vi "getSelfNode.vi"(8 "error in (no error)":errorcluster, 11 "Node in":refnum<class "Node.lvclass">) -> (0 "error out":errorcluster, 2 "selfNode":refnum<data-value>, 3 "Node out":refnum<class "Node.lvclass">)   [LabVIEW 2009, in "Node.lvclass"]
uses:
  Node.lvclass
  DataObj/DataObj.lvclass
  Node.lvclass/Node.ctl
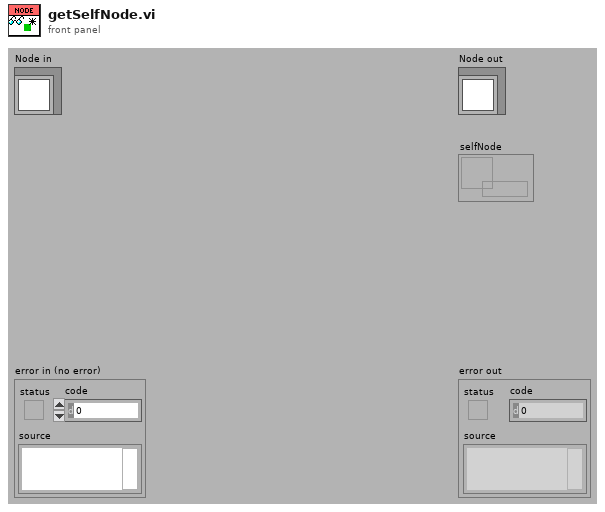
[diagram p1: front panel]
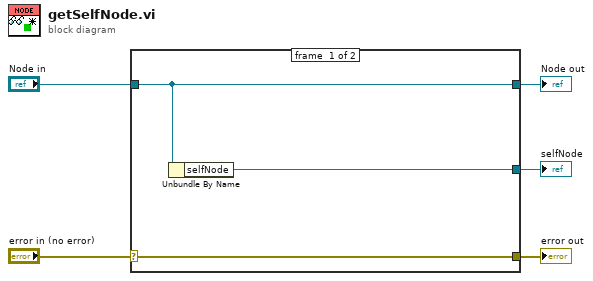
[diagram p0: block diagram]
diagram:
  n1 = case shown="No Error" "error in (no error)" {
    selector: "error in (no error)" -> [w8 w9]
    tunnel: [w8 w9] -> w4
    tunnel: [w7 w10] -> w2
    tunnel: "Node in" -> [w7 w10]
    tunnel: [w6 _] -> w1
    frame #0 {
      n2 = Unbundle By Name(w7) -> ("selfNode"=w6:refnum<data-value>)
    }
    frame #1 {
    }
  }
  "error out" <- w4
  "Node out" <- w2
  "selfNode" <- w1
